vi "methodeändern.vi"(2 "Methode":T1 {"FPGAPID"."proportional gain (Kc)" format="%.11g"; "FPGAPID"."integral gain (Kc*Ts/Ti)" format="%.11g"; "FPGAPID"."derivative gain (Kc*Td/Ts)" format="%.11g"; "FPGAFixp" format="%.14g"}, 3 "Namen":T2) -> (1 "Methode":T1 {"FPGAPID"."proportional gain (Kc)" format="%.11g"; "FPGAPID"."integral gain (Kc*Ts/Ti)" format="%.11g"; "FPGAPID"."derivative gain (Kc*Td/Ts)" format="%.11g"; "FPGAFixp" format="%.14g"})   [LabVIEW 2010]
panel:
  out "Methode":string
  in  "Int.Stop2":dbl
  in  "Int.Start2":dbl
  in  "Int.Stop1":dbl
  in  "Int.Start1":dbl
  in  "ZeitpktMS-2":dbl
  in  "ZeitpktMS-1":dbl
  in  "SetpointMPV":i32[](array[numeric]) min=1 max=6 step=1
  in  "ZeitpunkteMPV":dbl[](array[numeric])
  in  "Editor verlassen":bool
  out "Spannung Mach":fxp<+/-,16,4> format="%.14g"
  in  "Temperatur Mach":dbl
  out "Spannung Trap":fxp<+/-,16,4> format="%.14g"
  in  "Temperatur Trap":dbl
  out "langsameHeizungen":string[](array[string])
  out "HorstSPMod2B":string[](array[string])
  out "HorstSPMod2A":string[](array[string])
  out "HorstSPMod1":string[](array[string])
  out "HorstSPMod0":string[](array[string])
  out "DIOsSPMod0":string[](array[string])
  out "DIOsSPMod2A":string[](array[string])
  out "DIOsSPMod2B":string[](array[string])
  out "DIOsSPMod1":string[](array[string])
  in  "Zykluslängen [s]":dbl[](array[numeric])
  in  "MS-Daten?":bool
  in  "PIDs für \"träge\" Heizungen":T3(array[cluster])
  in  "TempMach2":dbl[](array[numeric])
  in  "ZeitpktMach2":dbl[](array[numeric])
  in  "TempMach1":dbl[](array[numeric])
  in  "ZeitpktMach1":dbl[](array[numeric])
  in  "FPGAFixp":fxp<+/-,16,4>[][](array[numeric]) format="%.14g"
  in  "ZeitpktFPGAFixp":dbl[](array[numeric])
  in  "FPGAPID":T4(array[cluster]) {"proportional gain (Kc)" format="%.11g"; "integral gain (Kc*Ts/Ti)" format="%.11g"; "derivative gain (Kc*Td/Ts)" format="%.11g"}
  in  "ZeitpktFPGAPID":dbl[](array[numeric])
  in  "FPGABoolesch":bool[][](array[boolean])
  in  "ZPktFPGABoolesch":dbl[](array[numeric])
  in  "LHHeizen?":bool[](array[boolean])
  in  "LangsameHeizungenSP":dbl[](array[numeric])
  in  "HorstSPMod2B":dbl[][](array[numeric])
  in  "HorstSPMod2A":dbl[][](array[numeric])
  in  "HorstSPMod1":dbl[][](array[numeric])
  in  "HorstSPMod0":dbl[][](array[numeric])
  in  "Mod2BHorstZeitpkt":dbl[](array[numeric])
  in  "Mod2AHorstZeitpkt":dbl[](array[numeric])
  in  "Mod1HorstZeitpkt":dbl[](array[numeric])
  in  "Mod0HorstZeitpkt":dbl[](array[numeric])
  in  "DIOsSPMod2B":bool[][](array[boolean])
  in  "DIOsSPMod2A":bool[][](array[boolean])
  in  "DIOsSPMod1":bool[][](array[boolean])
  in  "DIOsSPMod0":bool[][](array[boolean])
  in  "ZeitpktDIOsMod2B":dbl[](array[numeric])
  in  "ZeitpktDIOsMod2A":dbl[](array[numeric])
  in  "ZeitpktDIOsMod1":dbl[](array[numeric])
  in  "ZeitpktDIOsMod0":dbl[](array[numeric])
  # "GANZ WICHTIG: ALLE TABELLEN MÜSSEN MIT DEM ZEITPUNKT 0 BEGINNEN UND DÜRFEN NICHT ENDEN, BEVOR DER ZYKLUS BEENDET IST"
  # "Alle Zeiten und Zeitpunkte werden in Sekunden ausgedrückt;\nModul0, Modul1, Modul2A, Modul2B"
  # "Schaltverhalten der Digitalausgänge, geordnet nach Modulen:\nModul0"
  # "Schaltverhalten der Digitalausgänge, geordnet nach Modulen:\nModul1"
  # "Schaltverhalten der Digitalausgänge, geordnet nach Modulen:\nModul2A"
  # "Schaltverhalten der Digitalausgänge, geordnet nach Modulen:\nModul2B"
  # "Vorgaben für die digitalen Druck-/Flußregler, geordnet nach Modulen:\nModul0"
  # "Vorgaben für die digitalen Druck-/Flußregler, geordnet nach Modulen:\nModul1"
  # "Vorgaben für die digitalen Druck-/Flußregler, geordnet nach Modulen:\nModul2A"
  # "Vorgaben für die digitalen Druck-/Flußregler, geordnet nach Modulen:\nModul2B"
  # "\"Träge\" Heizungen: PID-Werte, Temperaturvorgaben und An/Aus"
  # "Boolesche Variablen zur Steuerung von Modul1"
  # "Servo1 kalt              Servo2 kalt            Trap1 heizen          Trap2 heizen          Mach1 heizen       Mach2 heizen"
  # "PID-Parameter für die \"schnellen\" Heizungen"
  # "Trap1                                            Trap2                                          Mach1                                         Mach2"
  # "Variablen zur Steuerung der \"schnellen\" Heizungen; Umrechnung: Temperatur in Spannung"
  # "U_Sollwert (Trap1)      U_Max (Trap1)           U_Widerst. (Trap1)    U_Sollwert (Trap2)      U_Max (Trap2)           U_Widerst. (Trap2)    U_Max (Mach1)         U_Max (Mach2)"
  # "Temperaturrampen für die Vorsäulen; die eingegebenen Punkte im (t-T)-Raum werden durch lineare Funktionen verbunden, jeweils definiert von Punkt zu Punkt"
  # "Sollen die Daten vom MS abgefragt werden? Wenn ja, zu welchen Zeitpunkten (im Zyklus1)"
  # "Stellung des Multipositionsventils; die Zeitpunkte beziehen sich auf den Zyklus von Modul0.\nDie Stellungen bezeichnen: 1. Standard3 - 2. Luftprobe - 3. Blank - 4. Standard1 - 5. Standard2 - 6. nicht belegt"
  # "Innerhalb welcher Zeitfenster soll der Probenfluß integriert werden?"
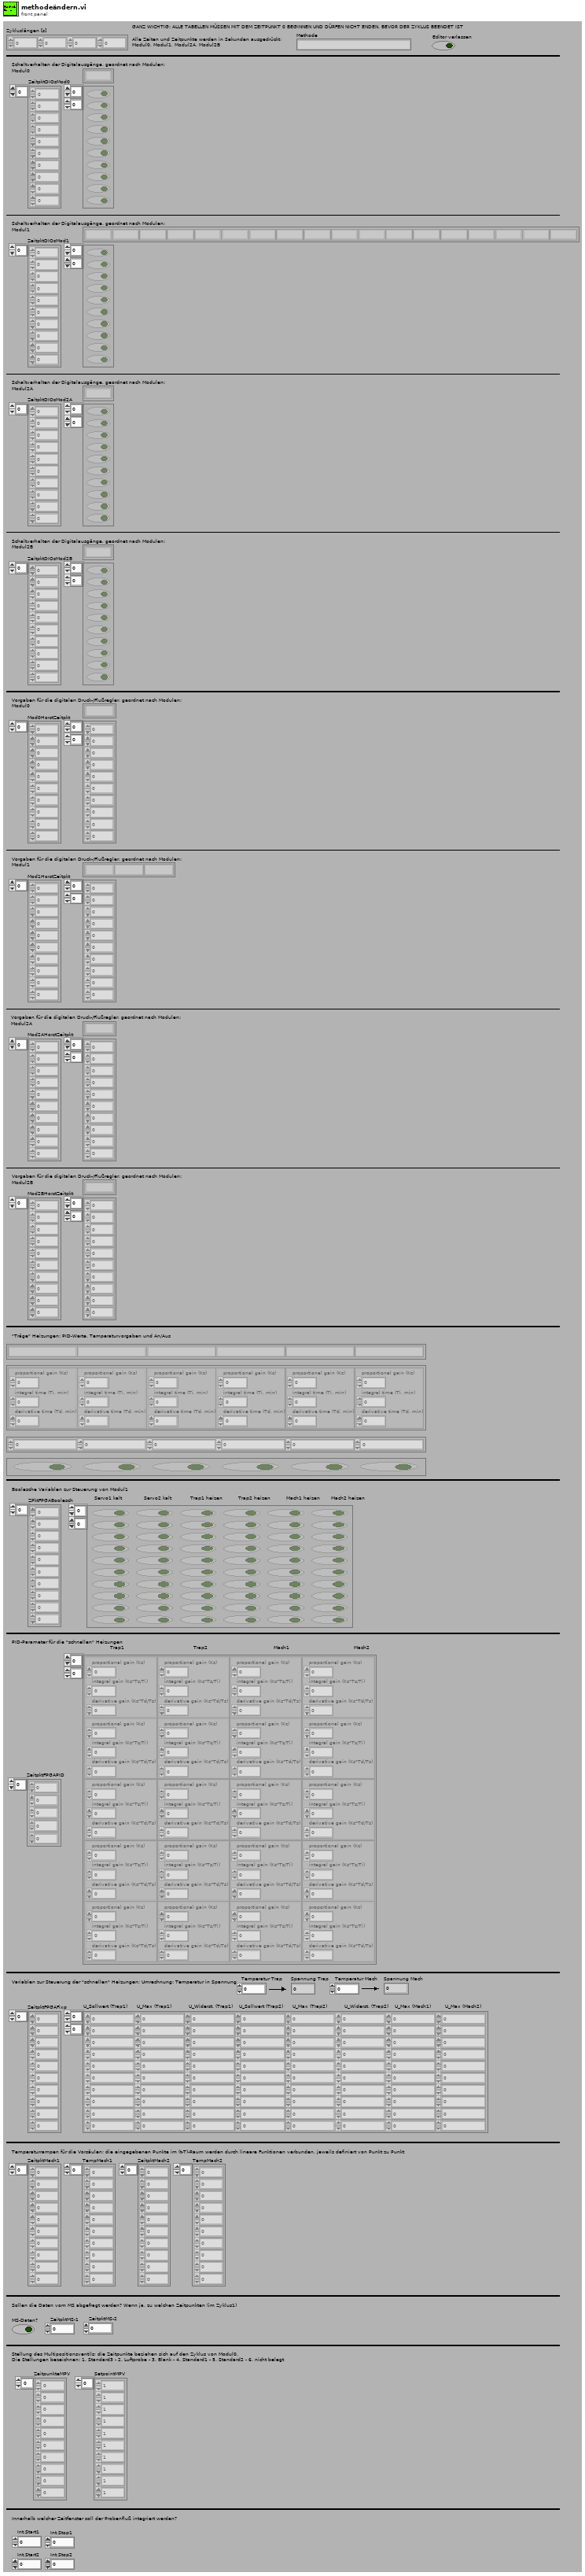
[diagram p1: front panel]
types:
  T1 = cluster{"Zykluslängen [s]":dbl[], "ZeitpktDIOsMod0":dbl[], "ZeitpktDIOsMod1":dbl[], "ZeitpktDIOsMod2A":dbl[], "ZeitpktDIOsMod2B":dbl[], "DIOsSPMod0":bool[][], "DIOsSPMod1":bool[][], "DIOsSPMod2A":bool[][], "DIOsSPMod2B":bool[][], "Mod0HorstZeitpkt":dbl[], "Mod1HorstZeitpkt":dbl[], "Mod2AHorstZeitpkt":dbl[], "Mod2BHorstZeitpkt":dbl[], "HorstSPMod0":dbl[][], "HorstSPMod1":dbl[][], "HorstSPMod2A":dbl[][], "HorstSPMod2B":dbl[][], "LangsameHeizungenSP":dbl[], "LHHeizen?":bool[], "ZPktFPGABoolesch":dbl[], "FPGABoolesch":bool[][], "ZeitpktFPGAPID":dbl[], "FPGAPID":cluster{"proportional gain (Kc)":fxp<+/-,16,8>, "integral gain (Kc*Ts/Ti)":fxp<+/-,16,8>, "derivative gain (Kc*Td/Ts)":fxp<+/-,16,8>}[][], "ZeitpktFPGAFixp":dbl[], "FPGAFixp":fxp<+/-,16,4>[][], "ZeitpktMach1":dbl[], "TempMach1":dbl[], "ZeitpktMach2":dbl[], "TempMach2":dbl[], "PIDs für \"träge\" Heizungen":cluster{"proportional gain (Kc)":dbl, "integral time (Ti, min)":dbl, "derivative time (Td, min)":dbl}[], "Zwangsbedingungen":dbl[][], "Dateien fürs MS schicken?":bool, "ZeitpunkteMPV":dbl[], "SPMPV":i32[], "ZeitpktMSa":dbl, "ZeitpktMSb":dbl, "Int.Start1":dbl, "Int.Stop1":dbl, "Int.Start2":dbl, "Int.Stop2":dbl, "Methodenname":string}
  T2 = cluster{"DIOsMod0Name":string[], "DIOsMod1Name":string[], "DIOsMod2AName":string[], "DIOsMod2BName":string[], "HorstMod0Name":string[], "HorstMod1Name":string[], "HorstMod2AName":string[], "HorstMod2BName":string[], string[]}
  T3 = cluster{"proportional gain (Kc)":dbl, "integral time (Ti, min)":dbl, "derivative time (Td, min)":dbl}[]
  T4 = cluster{"proportional gain (Kc)":fxp<+/-,16,8>, "integral gain (Kc*Ts/Ti)":fxp<+/-,16,8>, "derivative gain (Kc*Td/Ts)":fxp<+/-,16,8>}[][]
  T5 = cluster{"Zykluslängen [s]":dbl[], "ZeitpktDIOsMod0":dbl[], "ZeitpktDIOsMod1":dbl[], "ZeitpktDIOsMod2A":dbl[], "ZeitpktDIOsMod2B":dbl[], "DIOsSPMod0":bool[][], "DIOsSPMod1":bool[][], "DIOsSPMod2A":bool[][], "DIOsSPMod2B":bool[][], "Mod0HorstZeitpkt":dbl[], "Mod1HorstZeitpkt":dbl[], "Mod2AHorstZeitpkt":dbl[], "Mod2BHorstZeitpkt":dbl[], "HorstSPMod0":dbl[][], "HorstSPMod1":dbl[][], "HorstSPMod2A":dbl[][], "HorstSPMod2B":dbl[][], "LangsameHeizungenSP":dbl[], "LHHeizen?":bool[], "ZPktFPGABoolesch":dbl[], "FPGABoolesch":bool[][], "ZeitpktFPGAPID":dbl[], "FPGAPID":cluster{"proportional gain (Kc)":fxp<+/-,16,8>, "integral gain (Kc*Ts/Ti)":fxp<+/-,16,8>, "derivative gain (Kc*Td/Ts)":fxp<+/-,16,8>}[][], "ZeitpktFPGAFixp":dbl[], "FPGAFixp":fxp<+/-,16,4>[][], "ZeitpktMach1":dbl[], "TempMach1":dbl[], "ZeitpktMach2":dbl[], "TempMach2":dbl[], "PIDs für \"träge\" Heizungen":cluster{"proportional gain (Kc)":dbl, "integral time (Ti, min)":dbl, "derivative time (Td, min)":dbl}[], "Zwangsbedingungen":dbl[][], "MS-Daten?":bool, "ZeitpunkteMPV":dbl[], "SetpointMPV":i32[], "ZeitpktMS-1":dbl, "ZeitpktMS-2":dbl, "Int.Start1":dbl, "Int.Stop1":dbl, "Int.Start2":dbl, "Int.Stop2":dbl, "Methodenname":string}
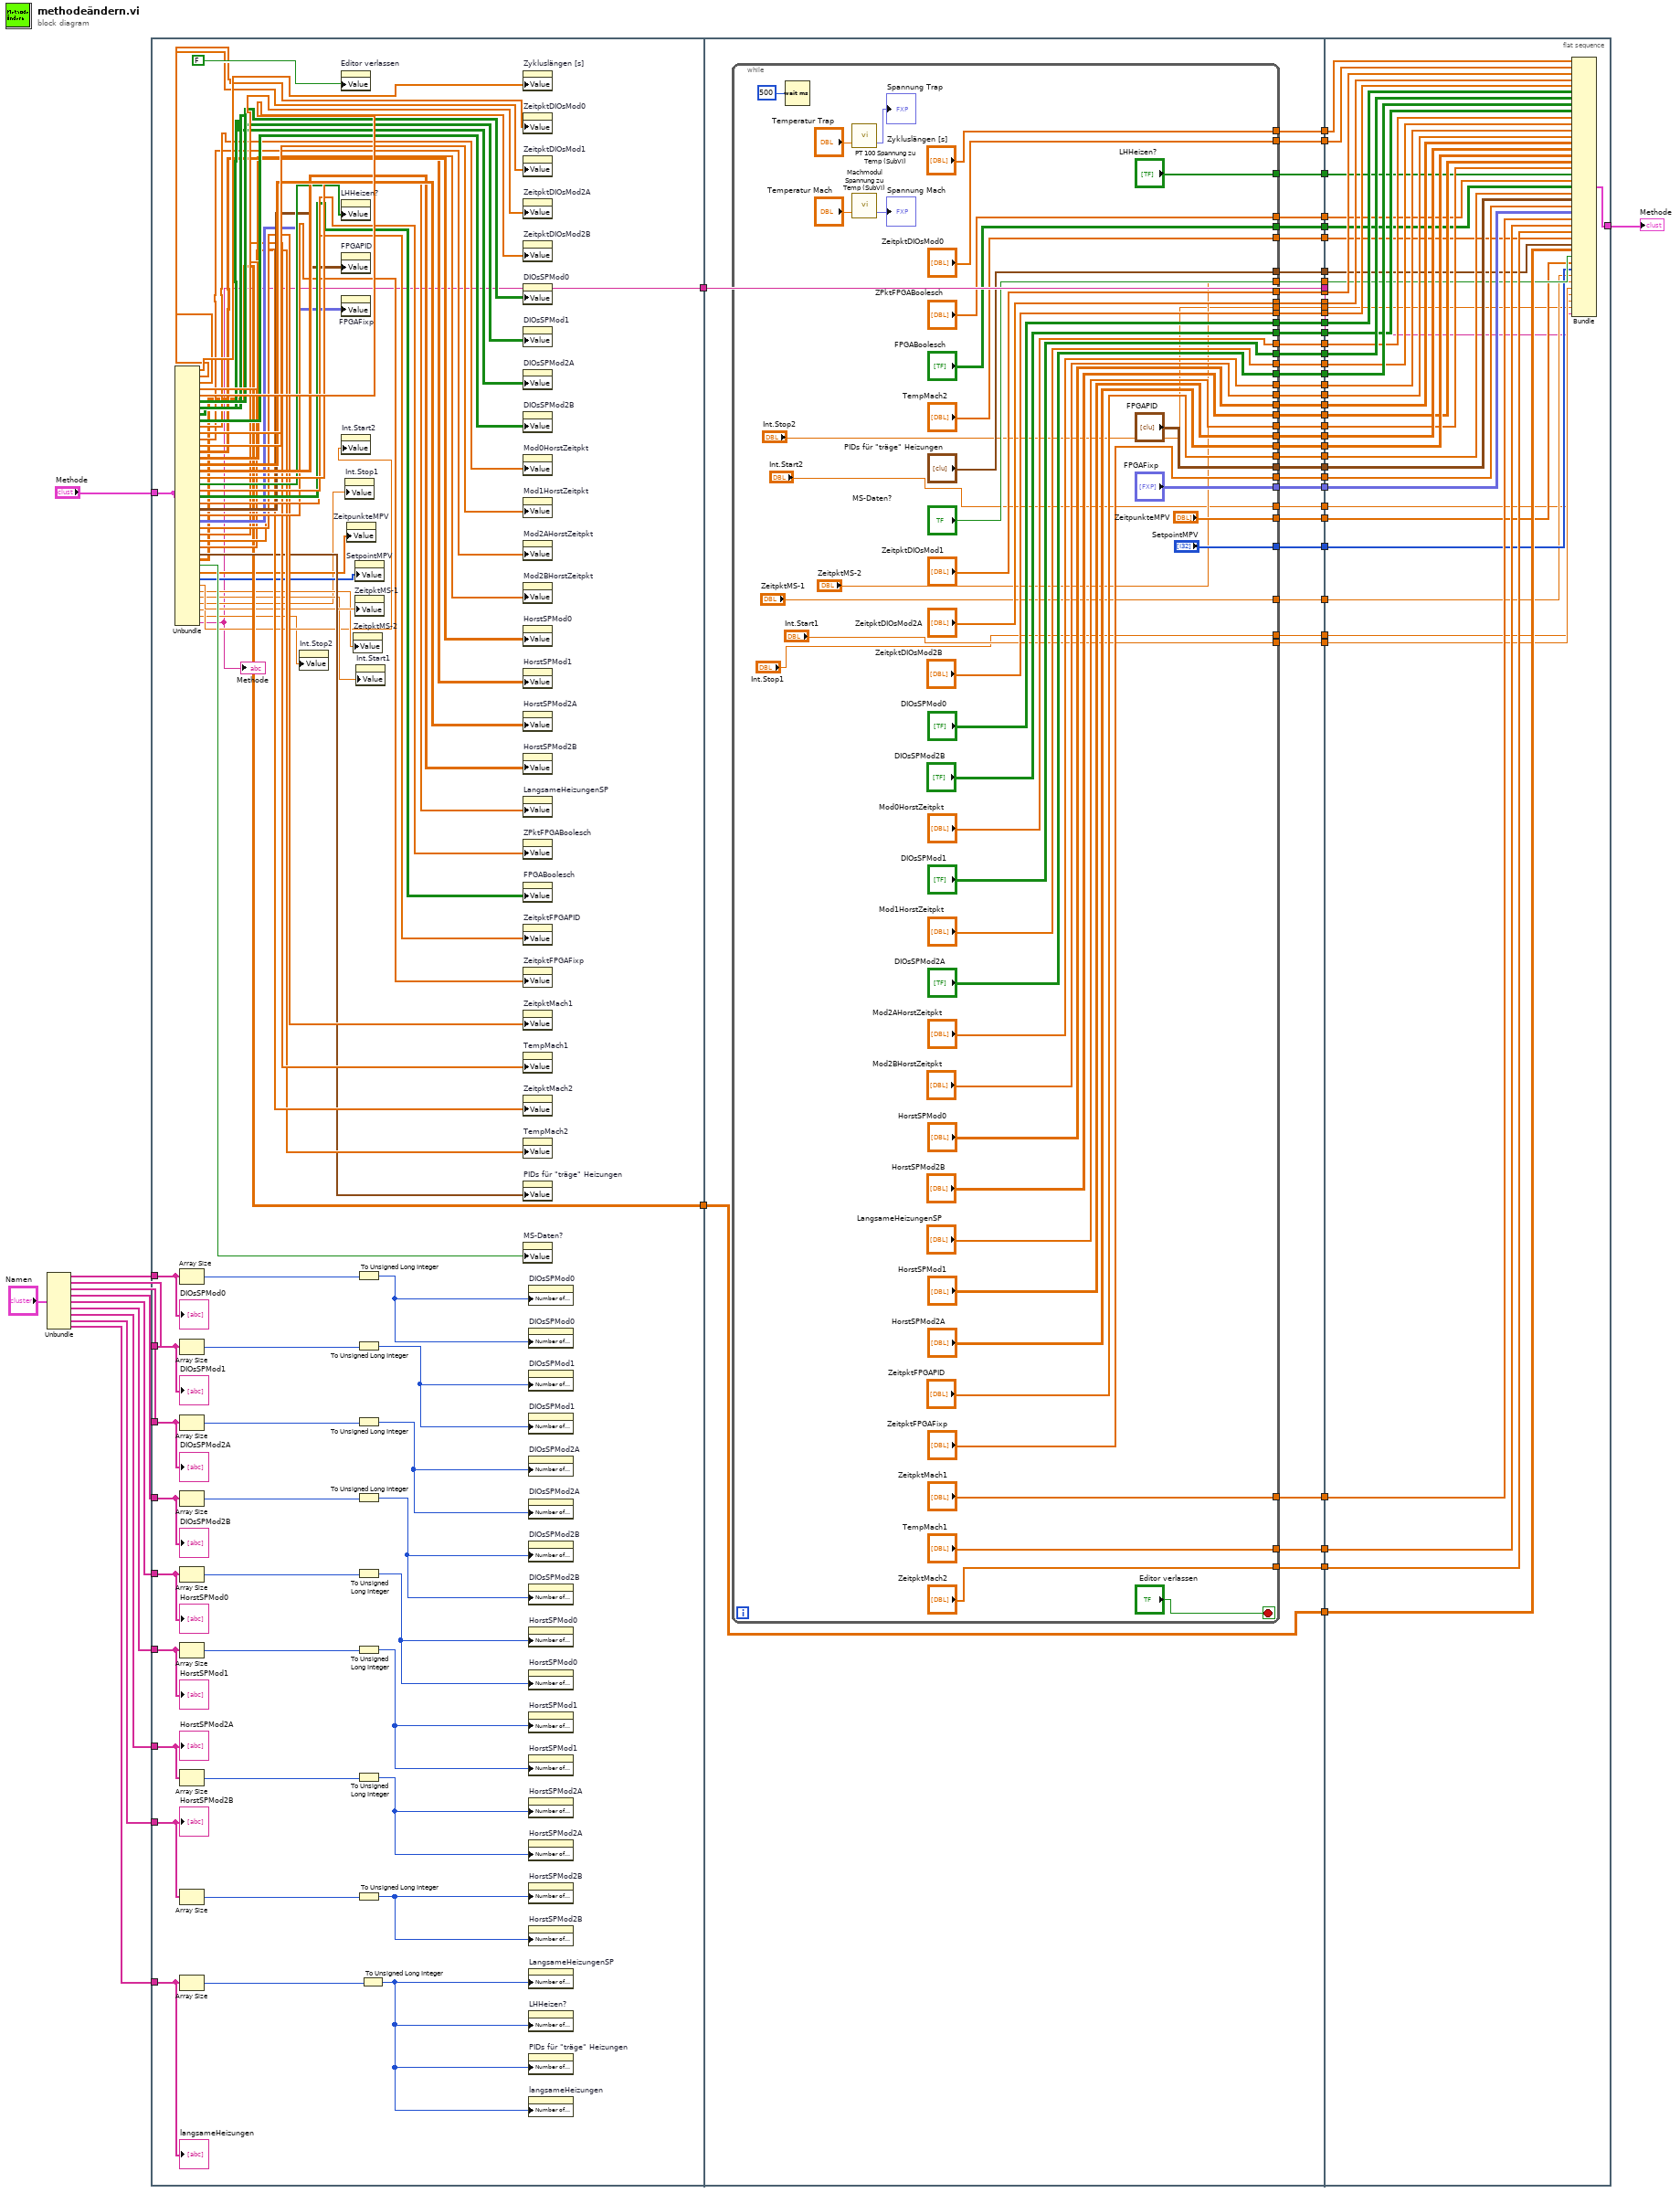
[diagram p0: block diagram]
diagram:
  n1 = Unbundle("Namen") -> ("DIOsMod0Name"=w21:string[], "DIOsMod1Name"=w20:string[], "DIOsMod2AName"=w19:string[], "DIOsMod2BName"=w18:string[], "HorstMod0Name"=w17:string[], "HorstMod1Name"=w16:string[], "HorstMod2AName"=w15:string[], "HorstMod2BName"=w14:string[], w13:string[])
  n2 = flat-sequence {
    tunnel: [w66] -> w25
    tunnel: w21 -> [w124]
    tunnel: w20 -> [w121]
    tunnel: w19 -> [w119]
    tunnel: w18 -> [w117]
    tunnel: w17 -> [w115]
    tunnel: w16 -> [w113]
    tunnel: w15 -> [w111]
    tunnel: w14 -> [w109]
    tunnel: w13 -> [w107]
    tunnel: [w97] -> _
    tunnel: "Methode" -> [w97]
    tunnel: [w56] -> w10
    tunnel: [w166] -> w55
    tunnel: [w165] -> w54
    tunnel: [w164] -> w53
    tunnel: [w163] -> w52
    tunnel: [w162] -> w51
    tunnel: [w161] -> w50
    tunnel: [w160] -> w49
    tunnel: [w159] -> w48
    tunnel: [w158] -> w47
    tunnel: [w157] -> w46
    tunnel: [w156] -> w45
    tunnel: [w155] -> w44
    tunnel: [w154] -> w43
    tunnel: [w153] -> w42
    tunnel: [w152] -> w41
    tunnel: [w151] -> w40
    tunnel: [w150] -> w39
    tunnel: [w149] -> w38
    tunnel: [w148] -> w37
    tunnel: [w147] -> w36
    tunnel: [w146] -> w35
    tunnel: [w145] -> w34
    tunnel: [w144] -> w33
    tunnel: [w143] -> w32
    tunnel: [w142] -> w31
    tunnel: [w141] -> w30
    tunnel: [w140] -> w29
    tunnel: [w139] -> w28
    tunnel: [w138] -> w27
    tunnel: [w137] -> w26
    tunnel: w25 -> [w137]
    tunnel: [w136] -> w24
    tunnel: [w135] -> w23
    tunnel: [w134] -> w11
    tunnel: w10 -> [w134]
    tunnel: [w133] -> w9
    tunnel: [w132] -> w8
    tunnel: [w131] -> w6
    tunnel: [w130] -> w5
    tunnel: [w129] -> w4
    tunnel: [w128] -> w3
    tunnel: [w127] -> w2
    tunnel: [w126] -> w1
    tunnel: w55 -> [w253]
    tunnel: w54 -> [w252]
    tunnel: w53 -> [w251]
    tunnel: w52 -> [w250]
    tunnel: w51 -> [w249]
    tunnel: w50 -> [w248]
    tunnel: w49 -> [w247]
    tunnel: w48 -> [w246]
    tunnel: w47 -> [w245]
    tunnel: w46 -> [w244]
    tunnel: w45 -> [w243]
    tunnel: w44 -> [w242]
    tunnel: w43 -> [w241]
    tunnel: w42 -> [w240]
    tunnel: w41 -> [w239]
    tunnel: w40 -> [w238]
    tunnel: w39 -> [w237]
    tunnel: w38 -> [w236]
    tunnel: w37 -> [w235]
    tunnel: w36 -> [w234]
    tunnel: w35 -> [w233]
    tunnel: w34 -> [w232]
    tunnel: w33 -> [w231]
    tunnel: w32 -> [w230]
    tunnel: w31 -> [w229]
    tunnel: w30 -> [w228]
    tunnel: w29 -> [w227]
    tunnel: w28 -> [w226]
    tunnel: w27 -> [w225]
    tunnel: w26 -> [w224]
    tunnel: w24 -> [w222]
    tunnel: w23 -> [w223]
    tunnel: w11 -> [w212]
    tunnel: w9 -> [w221]
    tunnel: w8 -> [w220]
    tunnel: [w219] -> w7
    tunnel: w6 -> [w218]
    tunnel: w5 -> [w217]
    tunnel: w4 -> [w216]
    tunnel: w3 -> [w215]
    tunnel: w2 -> [w214]
    tunnel: w1 -> [w213]
    frame #0 {
      n3 = Unbundle(w97) -> ("Zykluslängen [s]"=w96:dbl[], "ZeitpktDIOsMod0"=w95:dbl[], "ZeitpktDIOsMod1"=w94:dbl[], "ZeitpktDIOsMod2A"=w93:dbl[], "ZeitpktDIOsMod2B"=w92:dbl[], "DIOsSPMod0"=w91:bool[][], "DIOsSPMod1"=w90:bool[][], "DIOsSPMod2A"=w89:bool[][], "DIOsSPMod2B"=w88:bool[][], "Mod0HorstZeitpkt"=w87:dbl[], "Mod1HorstZeitpkt"=w86:dbl[], "Mod2AHorstZeitpkt"=w85:dbl[], "Mod2BHorstZeitpkt"=w84:dbl[], "HorstSPMod0"=w83:dbl[][], "HorstSPMod1"=w82:dbl[][], "HorstSPMod2A"=w81:dbl[][], "HorstSPMod2B"=w80:dbl[][], "LangsameHeizungenSP"=w79:dbl[], "LHHeizen?"=w78:bool[], "ZPktFPGABoolesch"=w77:dbl[], "FPGABoolesch"=w76:bool[][], "ZeitpktFPGAPID"=w75:dbl[], "FPGAPID"=w74:T4, "ZeitpktFPGAFixp"=w73:dbl[], "FPGAFixp"=w72:fxp<+/-,16,4>[][], "ZeitpktMach1"=w71:dbl[], "TempMach1"=w70:dbl[], "ZeitpktMach2"=w69:dbl[], "TempMach2"=w68:dbl[], "PIDs für \"träge\" Heizungen"=w67:T3, "Zwangsbedingungen"=w66:dbl[][], "Dateien fürs MS schicken?"=w65:bool, "ZeitpunkteMPV"=w64:dbl[], "SPMPV"=w63:i32[], "ZeitpktMSa"=w62:dbl, "ZeitpktMSb"=w61:dbl, "Int.Start1"=w60:dbl, "Int.Stop1"=w59:dbl, "Int.Start2"=w58:dbl, "Int.Stop2"=w57:dbl, "Methodenname"=w56:string)
      "Methode" <- w56
      n4 = Array Size(array=w124) -> (size(s)=w123:i32)
      n5 = Array Size(array=w121) -> (size(s)=w122:i32)
      n6 = Array Size(array=w119) -> (size(s)=w120:i32)
      n7 = Array Size(array=w117) -> (size(s)=w118:i32)
      n8 = Array Size(array=w115) -> (size(s)=w116:i32)
      n9 = Array Size(array=w113) -> (size(s)=w114:i32)
      n10 = Array Size(array=w111) -> (size(s)=w112:i32)
      n11 = Array Size(array=w109) -> (size(s)=w110:i32)
      n12 = Array Size(array=w107) -> (size(s)=w108:i32)
      n13 = property on="Int.Stop2" class="DigWert (strikt)"("Value"=w57) -> ()  [unwired: 2 in, 2 out]
      n14 = property on="Editor verlassen" class="Bool. (strikt)"("Value"=FALSE) -> ()  [unwired: 2 in, 2 out]
      n15 = property on="LHHeizen?" class="Arr (strikt)"("Value"=w78) -> ()  [unwired: 2 in, 2 out]
      n16 = property on="FPGAPID" class="Arr (strikt)"("Value"=w74) -> ()  [unwired: 2 in, 2 out]
      n17 = property on="FPGAFixp" class="Arr (strikt)"("Value"=w72) -> ()  [unwired: 2 in, 2 out]
      n18 = property on="Int.Start2" class="DigWert (strikt)"("Value"=w58) -> ()  [unwired: 2 in, 2 out]
      n19 = property on="Int.Stop1" class="DigWert (strikt)"("Value"=w59) -> ()  [unwired: 2 in, 2 out]
      n20 = property on="ZeitpunkteMPV" class="Arr (strikt)"("Value"=w64) -> ()  [unwired: 2 in, 2 out]
      n21 = property on="ZeitpktMS-2" class="DigWert (strikt)"("Value"=w61) -> ()  [unwired: 2 in, 2 out]
      n22 = property on="SetpointMPV" class="Arr (strikt)"("Value"=w63) -> ()  [unwired: 2 in, 2 out]
      n23 = property on="ZeitpktMS-1" class="DigWert (strikt)"("Value"=w62) -> ()  [unwired: 2 in, 2 out]
      n24 = property on="Int.Start1" class="DigWert (strikt)"("Value"=w60) -> ()  [unwired: 2 in, 2 out]
      n25 = To Unsigned Long Integer(number=w123) -> (unsigned 32bit integer=w106:u32)
      n26 = To Unsigned Long Integer(number=w122) -> (unsigned 32bit integer=w105:u32)
      n27 = To Unsigned Long Integer(number=w120) -> (unsigned 32bit integer=w104:u32)
      n28 = To Unsigned Long Integer(number=w118) -> (unsigned 32bit integer=w103:u32)
      n29 = To Unsigned Long Integer(number=w116) -> (unsigned 32bit integer=w102:u32)
      n30 = To Unsigned Long Integer(number=w114) -> (unsigned 32bit integer=w101:u32)
      n31 = To Unsigned Long Integer(number=w112) -> (unsigned 32bit integer=w100:u32)
      n32 = To Unsigned Long Integer(number=w110) -> (unsigned 32bit integer=w99:u32)
      n33 = To Unsigned Long Integer(number=w108) -> (unsigned 32bit integer=w98:u32)
      n34 = property on="Zykluslängen [s]" class="Arr (strikt)"("Value"=w96) -> ()  [unwired: 2 in, 2 out]
      n35 = property on="ZeitpktDIOsMod0" class="Arr (strikt)"("Value"=w95) -> ()  [unwired: 2 in, 2 out]
      n36 = property on="ZeitpktDIOsMod1" class="Arr (strikt)"("Value"=w94) -> ()  [unwired: 2 in, 2 out]
      n37 = property on="ZeitpktDIOsMod2A" class="Arr (strikt)"("Value"=w93) -> ()  [unwired: 2 in, 2 out]
      n38 = property on="ZeitpktDIOsMod2B" class="Arr (strikt)"("Value"=w92) -> ()  [unwired: 2 in, 2 out]
      n39 = property on="DIOsSPMod0" class="Arr (strikt)"("Value"=w91) -> ()  [unwired: 2 in, 2 out]
      n40 = property on="DIOsSPMod1" class="Arr (strikt)"("Value"=w90) -> ()  [unwired: 2 in, 2 out]
      n41 = property on="DIOsSPMod2A" class="Arr (strikt)"("Value"=w89) -> ()  [unwired: 2 in, 2 out]
      n42 = property on="DIOsSPMod2B" class="Arr (strikt)"("Value"=w88) -> ()  [unwired: 2 in, 2 out]
      n43 = property on="Mod0HorstZeitpkt" class="Arr (strikt)"("Value"=w87) -> ()  [unwired: 2 in, 2 out]
      n44 = property on="Mod1HorstZeitpkt" class="Arr (strikt)"("Value"=w86) -> ()  [unwired: 2 in, 2 out]
      n45 = property on="Mod2AHorstZeitpkt" class="Arr (strikt)"("Value"=w85) -> ()  [unwired: 2 in, 2 out]
      n46 = property on="Mod2BHorstZeitpkt" class="Arr (strikt)"("Value"=w84) -> ()  [unwired: 2 in, 2 out]
      n47 = property on="HorstSPMod0" class="Arr (strikt)"("Value"=w83) -> ()  [unwired: 2 in, 2 out]
      n48 = property on="HorstSPMod1" class="Arr (strikt)"("Value"=w82) -> ()  [unwired: 2 in, 2 out]
      n49 = property on="HorstSPMod2A" class="Arr (strikt)"("Value"=w81) -> ()  [unwired: 2 in, 2 out]
      n50 = property on="HorstSPMod2B" class="Arr (strikt)"("Value"=w80) -> ()  [unwired: 2 in, 2 out]
      n51 = property on="LangsameHeizungenSP" class="Arr (strikt)"("Value"=w79) -> ()  [unwired: 2 in, 2 out]
      n52 = property on="ZPktFPGABoolesch" class="Arr (strikt)"("Value"=w77) -> ()  [unwired: 2 in, 2 out]
      n53 = property on="FPGABoolesch" class="Arr (strikt)"("Value"=w76) -> ()  [unwired: 2 in, 2 out]
      n54 = property on="ZeitpktFPGAPID" class="Arr (strikt)"("Value"=w75) -> ()  [unwired: 2 in, 2 out]
      n55 = property on="ZeitpktFPGAFixp" class="Arr (strikt)"("Value"=w73) -> ()  [unwired: 2 in, 2 out]
      n56 = property on="ZeitpktMach1" class="Arr (strikt)"("Value"=w71) -> ()  [unwired: 2 in, 2 out]
      n57 = property on="TempMach1" class="Arr (strikt)"("Value"=w70) -> ()  [unwired: 2 in, 2 out]
      n58 = property on="ZeitpktMach2" class="Arr (strikt)"("Value"=w69) -> ()  [unwired: 2 in, 2 out]
      n59 = property on="TempMach2" class="Arr (strikt)"("Value"=w68) -> ()  [unwired: 2 in, 2 out]
      n60 = property on="PIDs für \"träge\" Heizungen" class="Arr (strikt)"("Value"=w67) -> ()  [unwired: 2 in, 2 out]
      n61 = property on="MS-Daten?" class="Bool. (strikt)"("Value"=w65) -> ()  [unwired: 2 in, 2 out]
      n62 = property on="DIOsSPMod0" class="Arr (strikt)"("Number of Columns"=w106) -> ()  [unwired: 2 in, 2 out]
      n63 = property on="DIOsSPMod0" class="Arr (strikt)"("Number of Columns"=w106) -> ()  [unwired: 2 in, 2 out]
      n64 = property on="DIOsSPMod1" class="Arr (strikt)"("Number of Columns"=w105) -> ()  [unwired: 2 in, 2 out]
      n65 = property on="DIOsSPMod1" class="Arr (strikt)"("Number of Columns"=w105) -> ()  [unwired: 2 in, 2 out]
      n66 = property on="DIOsSPMod2A" class="Arr (strikt)"("Number of Columns"=w104) -> ()  [unwired: 2 in, 2 out]
      n67 = property on="DIOsSPMod2A" class="Arr (strikt)"("Number of Columns"=w104) -> ()  [unwired: 2 in, 2 out]
      n68 = property on="DIOsSPMod2B" class="Arr (strikt)"("Number of Columns"=w103) -> ()  [unwired: 2 in, 2 out]
      n69 = property on="DIOsSPMod2B" class="Arr (strikt)"("Number of Columns"=w103) -> ()  [unwired: 2 in, 2 out]
      n70 = property on="HorstSPMod0" class="Arr (strikt)"("Number of Columns"=w102) -> ()  [unwired: 2 in, 2 out]
      n71 = property on="HorstSPMod0" class="Arr (strikt)"("Number of Columns"=w102) -> ()  [unwired: 2 in, 2 out]
      n72 = property on="HorstSPMod1" class="Arr (strikt)"("Number of Columns"=w101) -> ()  [unwired: 2 in, 2 out]
      n73 = property on="HorstSPMod1" class="Arr (strikt)"("Number of Columns"=w101) -> ()  [unwired: 2 in, 2 out]
      n74 = property on="HorstSPMod2A" class="Arr (strikt)"("Number of Columns"=w100) -> ()  [unwired: 2 in, 2 out]
      n75 = property on="HorstSPMod2A" class="Arr (strikt)"("Number of Columns"=w100) -> ()  [unwired: 2 in, 2 out]
      n76 = property on="HorstSPMod2B" class="Arr (strikt)"("Number of Columns"=w99) -> ()  [unwired: 2 in, 2 out]
      n77 = property on="HorstSPMod2B" class="Arr (strikt)"("Number of Columns"=w99) -> ()  [unwired: 2 in, 2 out]
      n78 = property on="LangsameHeizungenSP" class="Arr (strikt)"("Number of Columns"=w98) -> ()  [unwired: 2 in, 2 out]
      n79 = property on="LHHeizen?" class="Arr (strikt)"("Number of Columns"=w98) -> ()  [unwired: 2 in, 2 out]
      n80 = property on="PIDs für \"träge\" Heizungen" class="Arr (strikt)"("Number of Columns"=w98) -> ()  [unwired: 2 in, 2 out]
      n81 = property on="langsameHeizungen" class="Arr (strikt)"("Number of Columns"=w98) -> ()  [unwired: 2 in, 2 out]
      "DIOsSPMod1" <- w121
      "DIOsSPMod2B" <- w117
      "DIOsSPMod2A" <- w119
      "DIOsSPMod0" <- w124
      "HorstSPMod0" <- w115
      "HorstSPMod1" <- w113
      "HorstSPMod2A" <- w111
      "HorstSPMod2B" <- w109
      "langsameHeizungen" <- w107
    }
    frame #1 {
      n82 = while {
        tunnel: ["ZeitpktDIOsMod0"] -> w166
        tunnel: ["ZeitpktDIOsMod1"] -> w165
        tunnel: ["ZeitpktDIOsMod2A"] -> w164
        tunnel: ["ZeitpktDIOsMod2B"] -> w163
        tunnel: ["DIOsSPMod0"] -> w162
        tunnel: ["DIOsSPMod1"] -> w161
        tunnel: ["DIOsSPMod2A"] -> w160
        tunnel: ["DIOsSPMod2B"] -> w159
        tunnel: ["Mod0HorstZeitpkt"] -> w158
        tunnel: ["Mod1HorstZeitpkt"] -> w157
        tunnel: ["Mod2AHorstZeitpkt"] -> w156
        tunnel: ["Mod2BHorstZeitpkt"] -> w155
        tunnel: ["HorstSPMod0"] -> w154
        tunnel: ["HorstSPMod1"] -> w153
        tunnel: ["HorstSPMod2A"] -> w152
        tunnel: ["HorstSPMod2B"] -> w151
        tunnel: ["LangsameHeizungenSP"] -> w150
        tunnel: ["LHHeizen?"] -> w149
        tunnel: ["ZPktFPGABoolesch"] -> w148
        tunnel: ["FPGABoolesch"] -> w147
        tunnel: ["ZeitpktFPGAPID"] -> w146
        tunnel: ["FPGAPID"] -> w145
        tunnel: ["ZeitpktFPGAFixp"] -> w144
        tunnel: ["FPGAFixp"] -> w143
        tunnel: ["ZeitpktMach1"] -> w142
        tunnel: ["TempMach1"] -> w141
        tunnel: ["ZeitpktMach2"] -> w140
        tunnel: ["TempMach2"] -> w139
        tunnel: ["PIDs für \"träge\" Heizungen"] -> w138
        tunnel: ["MS-Daten?"] -> w136
        tunnel: ["Zykluslängen [s]"] -> w135
        tunnel: ["ZeitpunkteMPV"] -> w133
        tunnel: ["SetpointMPV"] -> w132
        tunnel: ["ZeitpktMS-1"] -> w131
        tunnel: ["ZeitpktMS-2"] -> w130
        tunnel: ["Int.Start1"] -> w129
        tunnel: ["Int.Stop1"] -> w128
        tunnel: ["Int.Start2"] -> w127
        tunnel: ["Int.Stop2"] -> w126
        stop <- "Editor verlassen" stop-if-true
        n83 = Wait (ms)(milliseconds to wait=u32 500 ("Zu wartende ms")) -> ()  [unwired: 1 out]
        n84 = call "PT 100 Spannung zu Temp (SubVI).vi"("Temp PT 100 soll"="Temperatur Trap") -> ("U soll"=→"Spannung Trap":fxp<+/-,16,4>)  [unwired: 1 in, 1 out]
        n85 = call "Machmodul Spannung zu Temp (SubVI).vi"("Temp PT 100 soll"="Temperatur Mach") -> ("U soll"=→"Spannung Mach":fxp<+/-,16,4>)  [unwired: 1 in, 1 out]
      }
    }
    frame #2 {
      n86 = Bundle("Zykluslängen [s]"=w223, "ZeitpktDIOsMod0"=w253, "ZeitpktDIOsMod1"=w252, "ZeitpktDIOsMod2A"=w251, "ZeitpktDIOsMod2B"=w250, "DIOsSPMod0"=w249, "DIOsSPMod1"=w248, "DIOsSPMod2A"=w247, "DIOsSPMod2B"=w246, "Mod0HorstZeitpkt"=w245, "Mod1HorstZeitpkt"=w244, "Mod2AHorstZeitpkt"=w243, "Mod2BHorstZeitpkt"=w242, "HorstSPMod0"=w241, "HorstSPMod1"=w240, "HorstSPMod2A"=w239, "HorstSPMod2B"=w238, "LangsameHeizungenSP"=w237, "LHHeizen?"=w236, "ZPktFPGABoolesch"=w235, "FPGABoolesch"=w234, "ZeitpktFPGAPID"=w233, "FPGAPID"=w232, "ZeitpktFPGAFixp"=w231, "FPGAFixp"=w230, "ZeitpktMach1"=w229, "TempMach1"=w228, "ZeitpktMach2"=w227, "TempMach2"=w226, "PIDs für \"träge\" Heizungen"=w225, "Zwangsbedingungen"=w224, "MS-Daten?"=w222, "ZeitpunkteMPV"=w221, "SetpointMPV"=w220, "ZeitpktMS-1"=w218, "ZeitpktMS-2"=w217, "Int.Start1"=w216, "Int.Stop1"=w215, "Int.Start2"=w214, "Int.Stop2"=w213, "Methodenname"=w212) -> (w219:T5)  [unwired: 1 in]
    }
  }
  "Methode" <- w7
